vi "Performance Test.vi"() -> ()   [LabVIEW 2021]
uses:
  <vilib>/Platform/TimedLoop/XDataNode/timing_clust.ctl
  <vilib>/Platform/TimedLoop/XDataNode/nitl_modes.ctl
  <vilib>/Platform/TimedLoop/XDataNode/wakeup.ctl
  1483eb5a-b5ac-4c0e-b74c-86c7137b2fd6.vi
  12cff863-7c17-483c-86ff-8b13899d7475.vi
  e1d05524-1b70-4109-b7da-ed5891de264b.vi
  929446f6-8a14-498e-9777-57eb22ff0df0.vi
  225441bf-869c-4d3f-a299-9c2de2de7507.vi
  b5d6512a-7382-4e79-b500-a81ead5716f2.vi
  eb2f4adc-c9c5-4356-9fb7-2e53ab499b8d.vi
  07197f74-83c7-460d-bb9d-2f7d38ffd2b9.vi
  21ba3f00-3ca1-4894-b9dd-4e112eabbaa9.vi
  def0a351-4179-4148-9177-b840eaa38f15.vi
  628c775d-4bce-4786-9b92-72b6beaba665.vi
  f43c1be1-ffa2-434e-887c-5abbb6a0f76a.vi
  b8af7206-5871-4d3b-9378-5cfe84a082f3.vi
  c2d7da70-2e27-4f49-958b-30f48dc9c665.vi
  ac27c80e-df74-46b0-978f-8f0f89081651.vi
  1483eb5a-b5ac-4c0e-b74c-86c7137b2fd6.vi/bd07d5d9-1209-45ad-b636-9e9ab86132fb.vi
  SubVIs/Check Error.vi
  SubVIs/Get dll Path.vi
  SubVIs/Get Element Write Position.vi
  SubVIs/Notify Of New Write.vi
  SubVIs/Wait For N Elements Available.vi
  SubVIs/Get Element Read Position.vi
  SubVIs/Set Element Read Position.vi
  225441bf-869c-4d3f-a299-9c2de2de7507.vi/49b3dd2d-4579-4089-b72e-3f0875c862f2.vi
  21ba3f00-3ca1-4894-b9dd-4e112eabbaa9.vi/49b3dd2d-4579-4089-b72e-3f0875c862f2.vi
  f43c1be1-ffa2-434e-887c-5abbb6a0f76a.vi/49b3dd2d-4579-4089-b72e-3f0875c862f2.vi
  <vilib>/Utility/error.llb/Trim Whitespace.vi
  <vilib>/string/Create NI GUID.vi
  SubVIs/Get Element Description Variant.vi
  <vilib>/Utility/error.llb/Error Cluster From Error Code.vi
  SubVIs/Get Element Info Variant.vi
  <vilib>/Platform/TimedLoop/XDataNode/XDataNode.xnode
  <vilib>/Platform/TimedLoop/XDataNode/XDNodeRunTimeDep.lvlib
  CIF_NI_CIPC.lvlib
panel:
  out "avg write double":dbl
  out "max write double":dbl
  out "avg read double no writer":dbl
  out "max read double no writer":dbl
  out "avg read double":dbl
  out "max read double":dbl
  in  "stop":bool
  out "avg read large array":dbl
  out "max read large array":dbl
  out "pass":bool
  out "error out":errorcluster
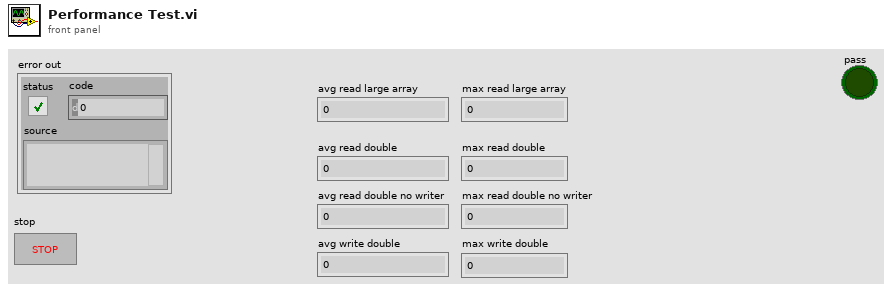
[diagram p1: front panel]
types:
  T1 = typedef "XDNodeRunTimeDep.lvlib/timing_clust.ctl" = cluster{"Expected End [f-1]":u64, "Actual End [f-1]":u64, "Finished Late? [f-1]":bool, "Expected End [i-1]":u64, "Actual End [i-1]":u64, "Finished Late? [i-1]":bool, "Expected Start [i]":u64, "Actual Start [i]":u64, "Expected Start [f]":u64, "Actual Start [f]":u64, "Source Name":string, "Structure Name":string, "Period":i64, "Deadline":i64, "Offset":i64, "Start":i64, "Priority":i32, "Timeout":i32, "Mode":T2, "Wakeup Reason":T3, "Error":errorcluster, "Source Type":string, "Secondary Source Type":string, "Global End Time":u64, "Global Start Time":u64, "Frame Duration":u64, "Iteration Duration":u64, "Assigned CPU":i32, "I/O Scan Engine Mode":u32}
  T2 = typedef "XDNodeRunTimeDep.lvlib/nitl_modes.ctl" = enum32{"No Change", "Process missed periods, maintain original phase", "Discard missed periods, maintain original phase", "Process missed periods, ignore original phase", "Discard missed periods, ignore original phase"}
  T3 = typedef "XDNodeRunTimeDep.lvlib/wakeup.ctl" = enum32{"Normal", "Aborted", "Asynchronous wakeup", "Timing source error", "Timed loop error", "Timeout"}
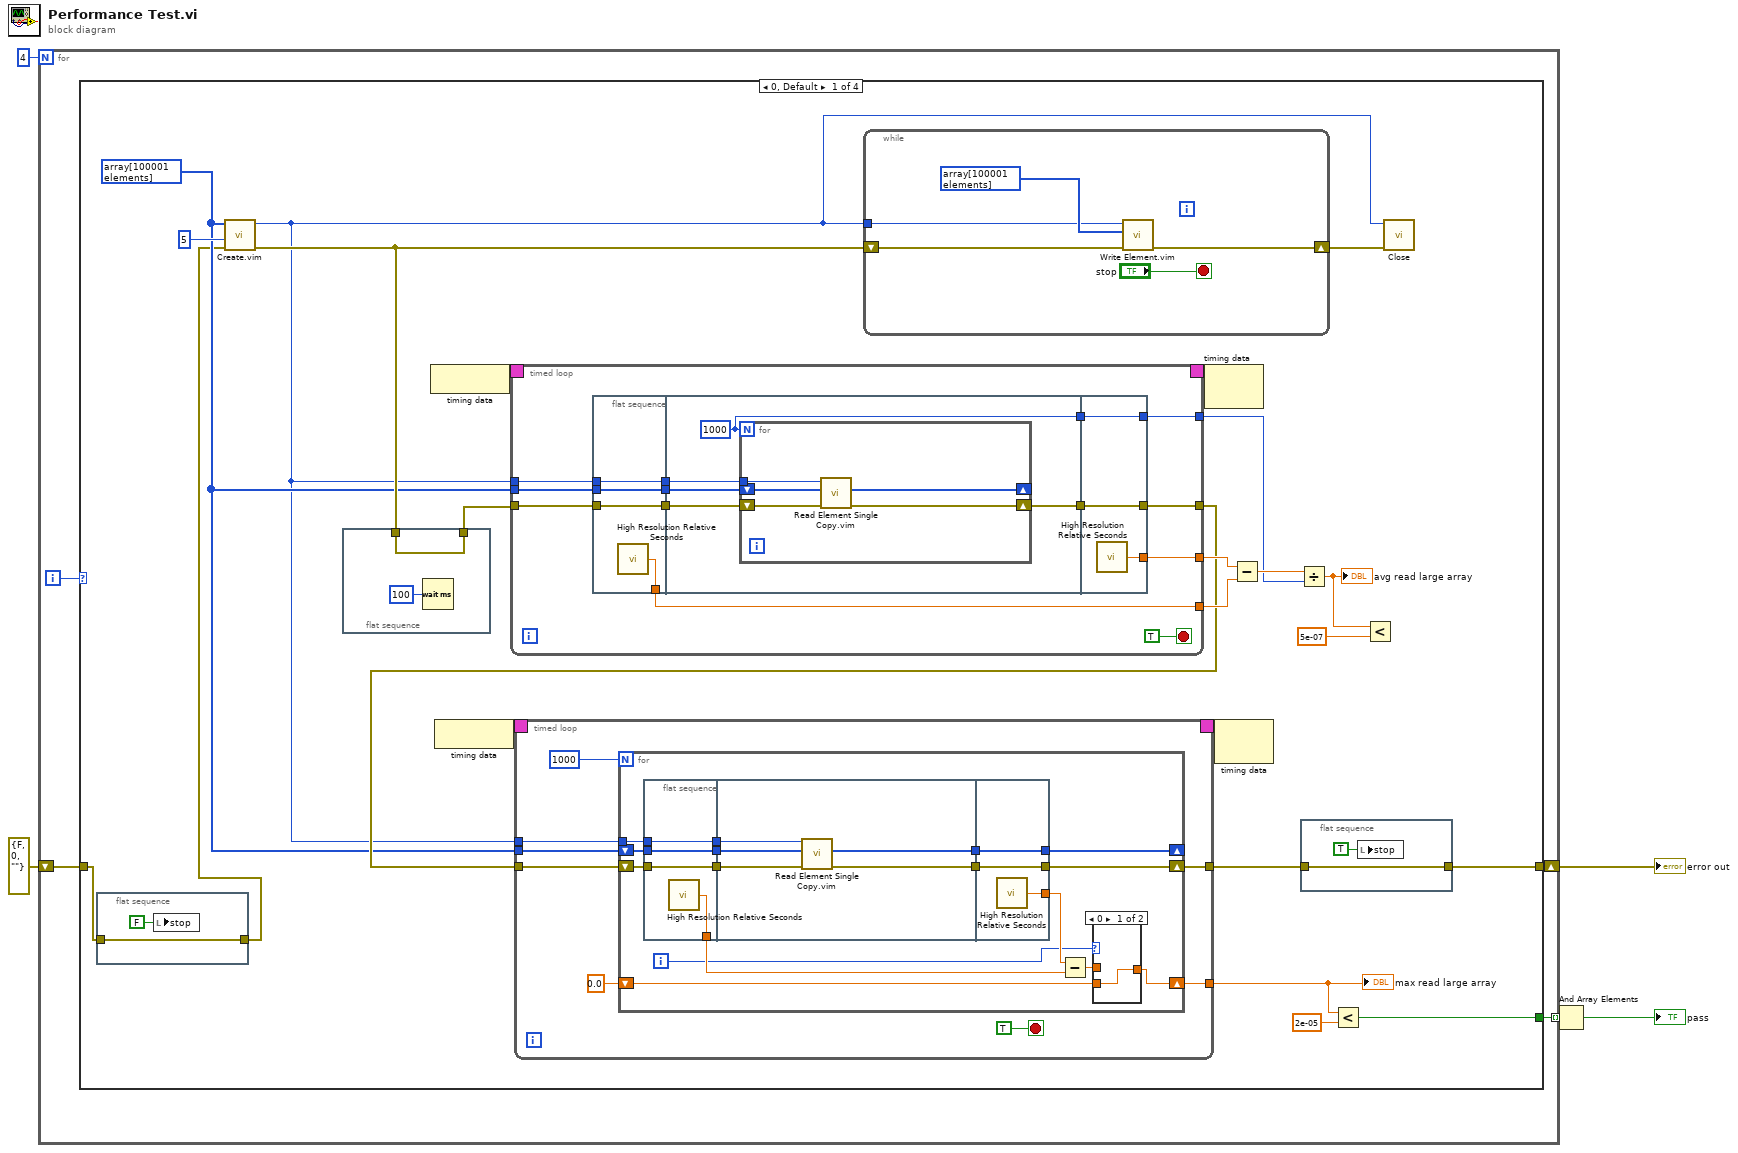
[diagram p0: block diagram]
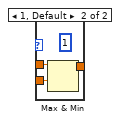
[diagram p2: hidden frame]
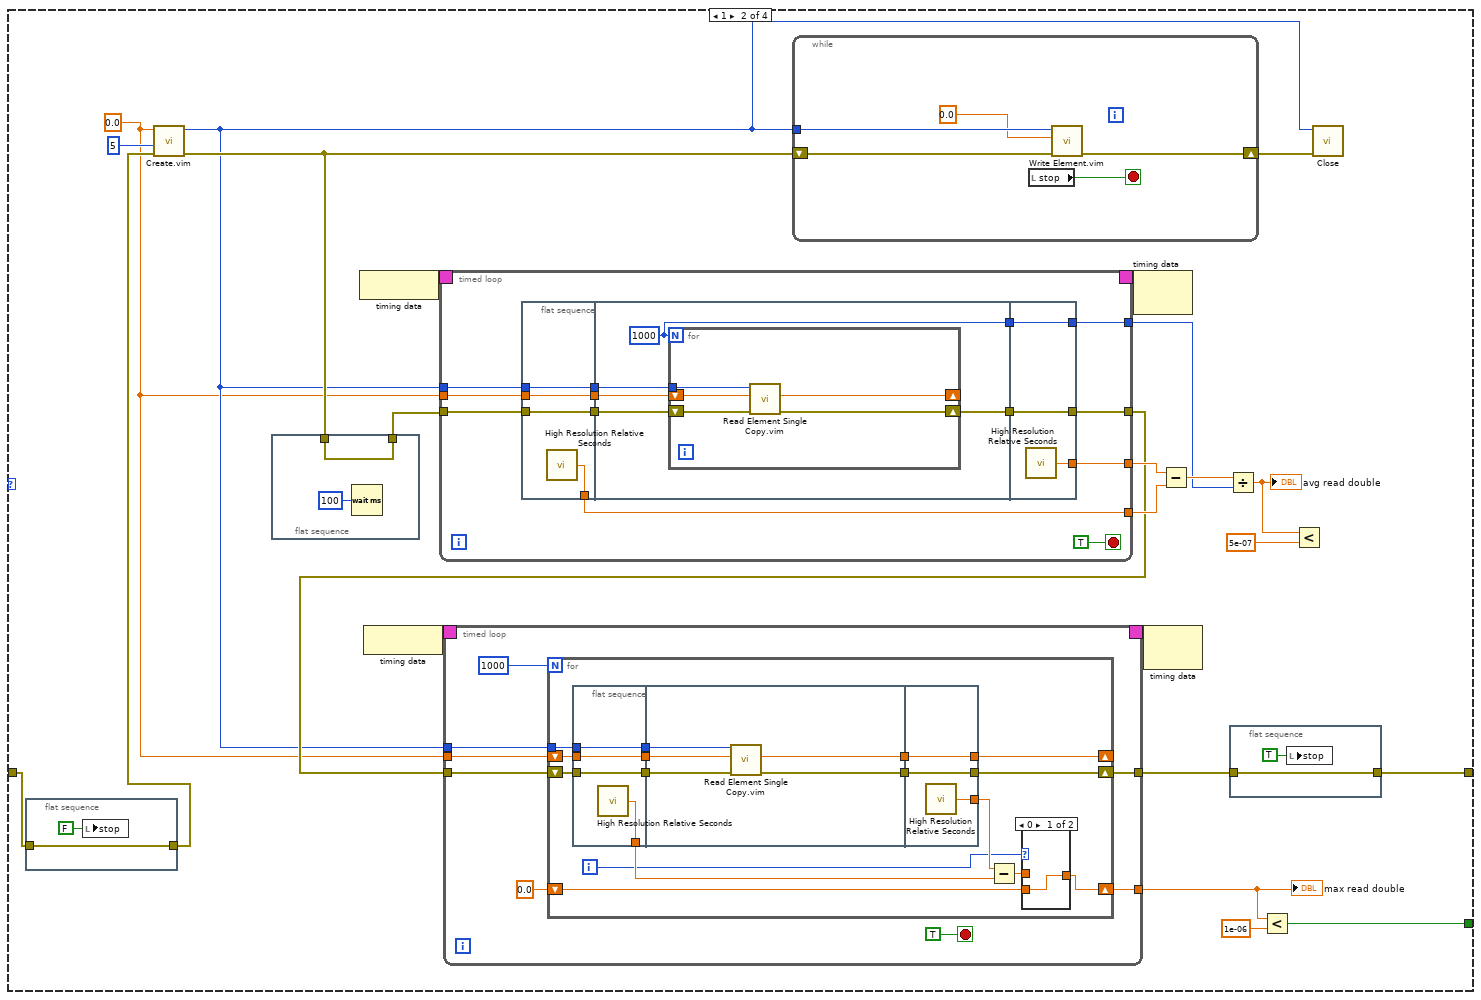
[diagram p3: hidden frame]
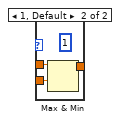
[diagram p4: hidden frame]
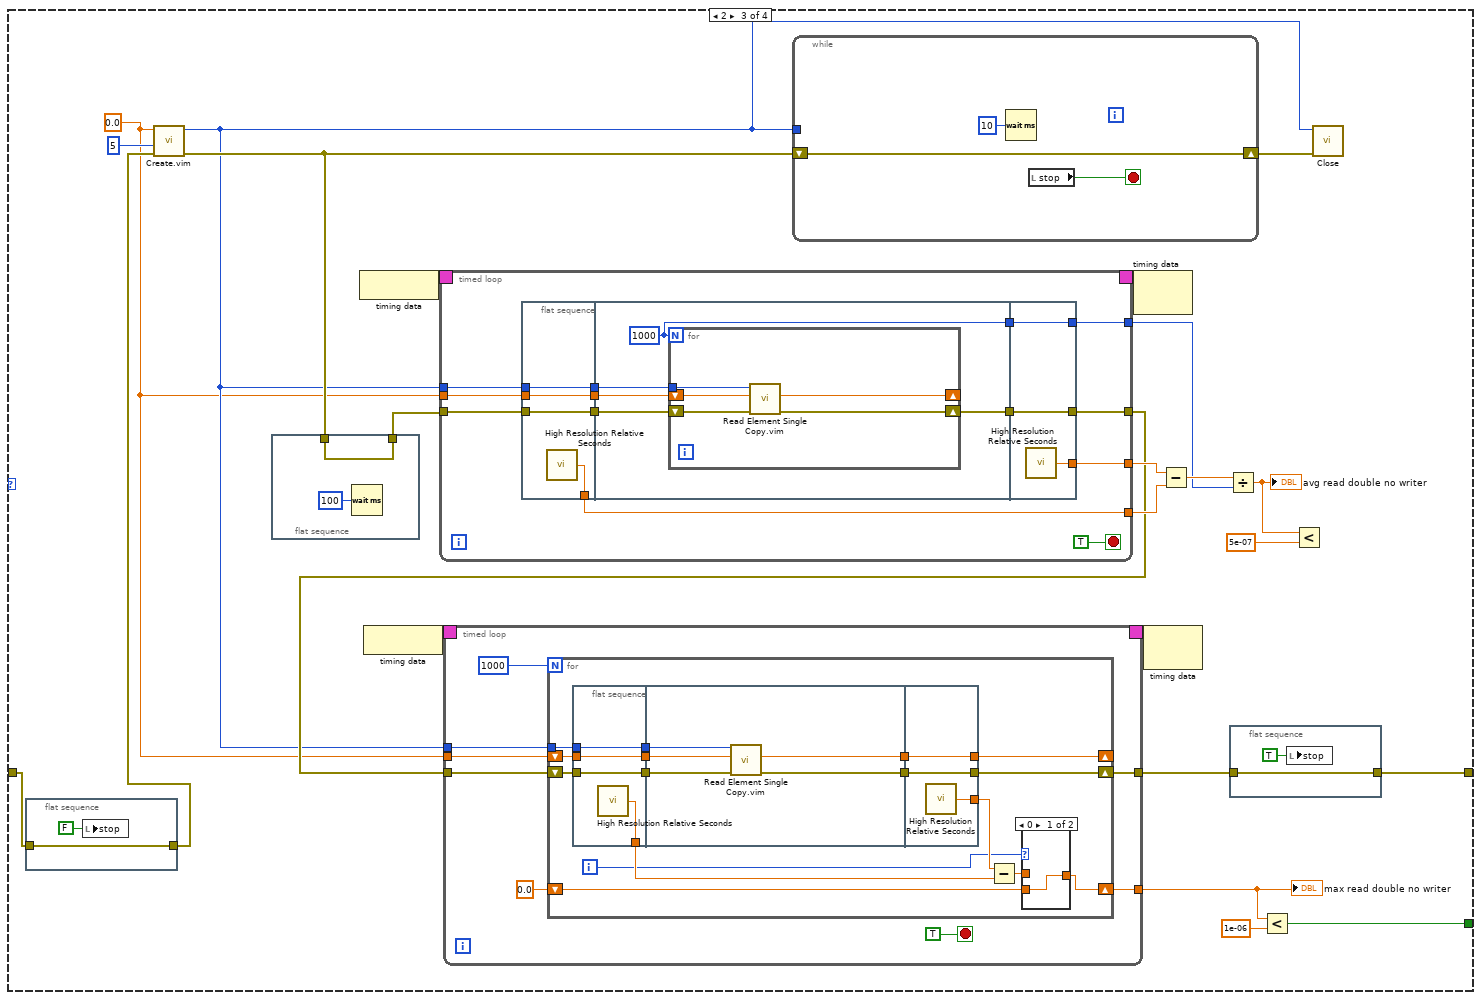
[diagram p5: hidden frame]
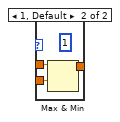
[diagram p6: hidden frame]
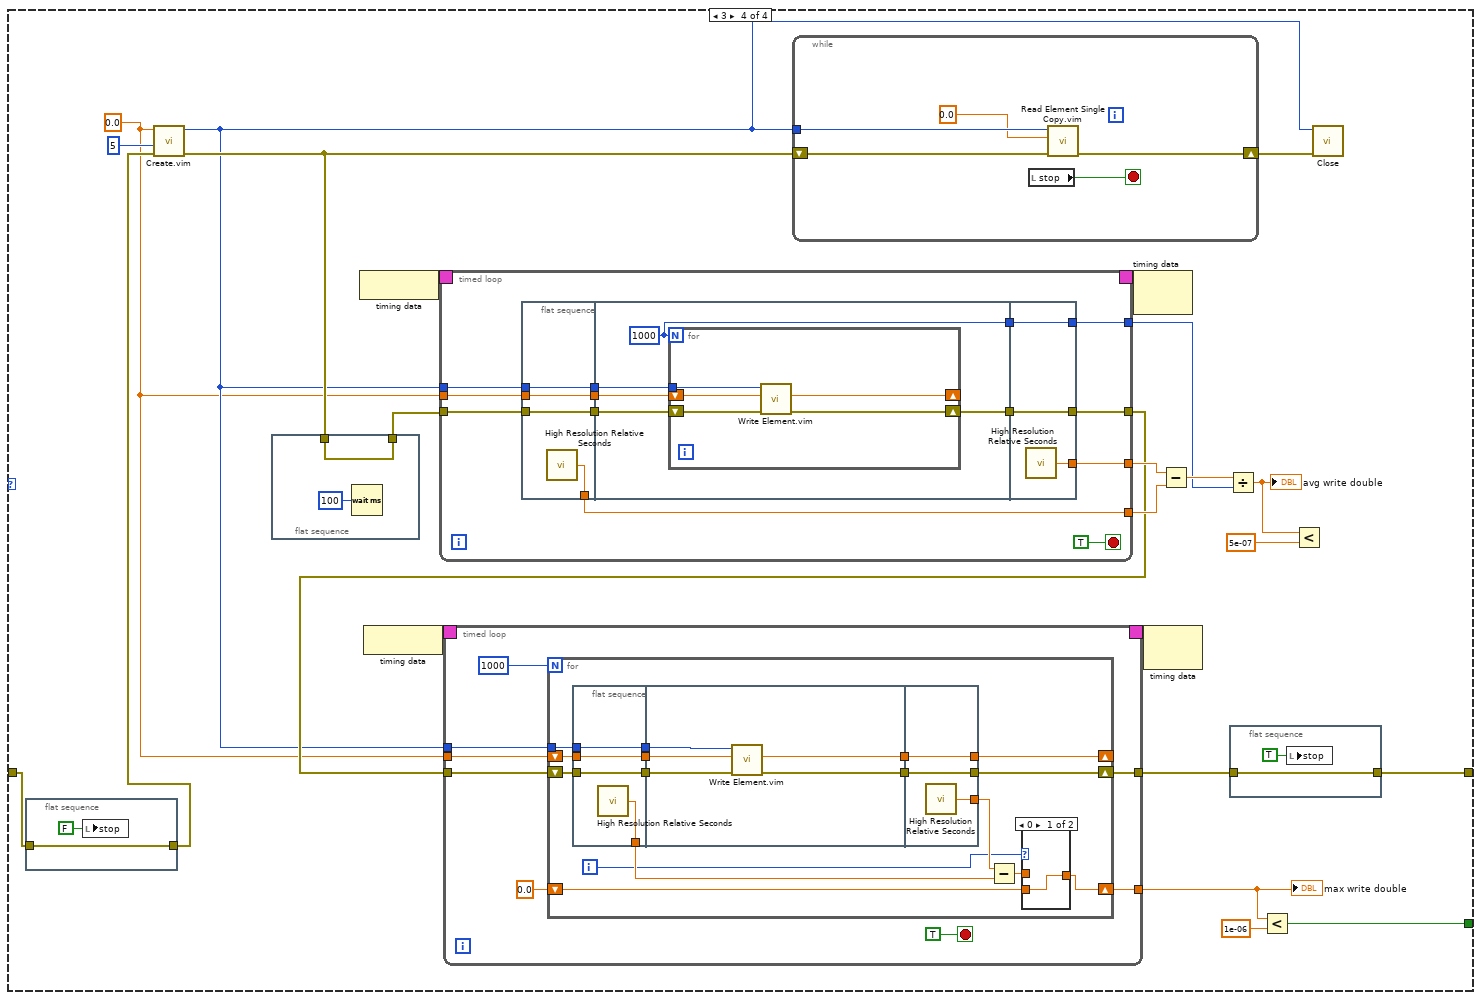
[diagram p7: hidden frame]
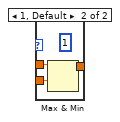
[diagram p8: hidden frame]
diagram:
  n1 = for {
    N: 4 -> [_]
    tunnel: [w9] -> w3 mode=indexing
    shift-right: [w8] -> w5
    shift-left: errorcluster {"status"=FALSE, "code"=0, "source"=""} ("error out") -> [w6]
    i -> [w7]
    n2 = case shown="0, Default" w7 {
      tunnel: [w20 w133 w246 w357] -> w9
      tunnel: [w12 w126 w239 w350] -> w8
      tunnel: w6 -> [w11 w125 w238 w349]
      frame 0, Default {
        w16 = u8[] array[100001 elements] ("U8 Data")
        n3 = flat-sequence {
          tunnel: w11 -> [w35]
          tunnel: [w35] -> w10
          frame #0 {
            n4 = local write "stop"(FALSE ("stop")) -> ()
          }
        }
        n5 = call "Create.vim"("error in (no error)"=w10, "Buffer Size N (2^N)"=u32 5, "Data Type"=w16) -> ("error out"=w17:errorcluster, "CIPC Reference"=w14:u64)  [unwired: 5 in, 2 out]
        n6 = flat-sequence {
          tunnel: w17 -> [w39]
          tunnel: [w39] -> w19
          frame #0 {
            n7 = Wait (ms)(milliseconds to wait=u32 100) -> ()  [unwired: 1 out]
          }
        }
        n8 = node-c288() -> (w33:T1)
        n9 = node-c288() -> (w31:T1)
        n10 = timed-loop {
          timing: w33 -> [_]
          timing-out: [_] -> w32
          tunnel: w14 -> [w91]
          tunnel: w19 -> [w101]
          tunnel: [w98] -> w25
          tunnel: [w96] -> w29
          tunnel: [w95] -> w28
          tunnel: [w94] -> w26
          tunnel: w16 -> [w89]
          stop <- TRUE stop-if-true
          n11 = flat-sequence {
            tunnel: w101 -> [w105]
            tunnel: [w105] -> w99
            tunnel: [w104] -> w95
            tunnel: [w103] -> w92
            tunnel: w91 -> [w103]
            tunnel: [w102] -> w90
            tunnel: w89 -> [w102]
            tunnel: w99 -> [w110]
            tunnel: [w109] -> w97
            tunnel: [w108] -> w93
            tunnel: w92 -> [w107]
            tunnel: w90 -> [w106]
            tunnel: [w118] -> w98
            tunnel: w97 -> [w118]
            tunnel: [w117] -> w96
            tunnel: [w116] -> w94
            tunnel: w93 -> [w116]
            frame #0 {
              n12 = call <vilib>:"High Resolution Relative Seconds.vi"() -> ("relative seconds"=w104:dbl)
            }
            frame #1 {
              w108 = 1000
              n13 = for {
                N: w108 -> [_]
                shift-right: [w113] -> _
                shift-left: w106 -> [w111]
                shift-right: [w114] -> w109
                shift-left: w110 -> [w115]
                tunnel: w107 -> [w112]
                n14 = call "Read Element Single Copy.vim"("error in (no error)"=w115, "Data in"=w111, "CIPC Reference"=w112) -> ("error out"=w114:errorcluster, "Data out"=w113:u8[])  [unwired: 5 in, 2 out]
              }
            }
            frame #2 {
              n15 = call <vilib>:"High Resolution Relative Seconds.vi"() -> ("relative seconds"=w117:dbl)
            }
          }
        }
        n16 = timed-loop {
          timing: w31 -> [_]
          timing-out: [_] -> w30
          tunnel: w25 -> [w52]
          tunnel: [w50] -> w13
          tunnel: [w47] -> w22
          tunnel: w16 -> [w46]
          tunnel: w14 -> [w45]
          stop <- TRUE stop-if-true
          n17 = for {
            N: 1000 -> [_]
            shift-right: [w63] -> _
            shift-left: w46 -> [w65]
            shift-right: [w62] -> w50
            shift-left: w52 -> [w64]
            shift-right: [w57] -> w47
            shift-left: 0.0 -> [w58]
            tunnel: w45 -> [w53]
            i -> [w56]
            n18 = flat-sequence {
              tunnel: w64 -> [w75]
              tunnel: w65 -> [w76]
              tunnel: [w76] -> w68
              tunnel: [w75] -> w67
              tunnel: [w74] -> w60
              tunnel: [w73] -> w54
              tunnel: w53 -> [w73]
              tunnel: w68 -> [w81]
              tunnel: w67 -> [w80]
              tunnel: [w79] -> w66
              tunnel: [w77] -> w55
              tunnel: w54 -> [w78]
              tunnel: [w84] -> w63
              tunnel: w66 -> [w84]
              tunnel: [w83] -> w62
              tunnel: [w82] -> w61
              tunnel: w55 -> [w83]
              frame #0 {
                n19 = call <vilib>:"High Resolution Relative Seconds.vi"() -> ("relative seconds"=w74:dbl)
              }
              frame #1 {
                n20 = call "Read Element Single Copy.vim"("error in (no error)"=w80, "Data in"=w81, "CIPC Reference"=w78) -> ("error out"=w77:errorcluster, "Data out"=w79:u8[])  [unwired: 5 in, 2 out]
              }
              frame #2 {
                n21 = call <vilib>:"High Resolution Relative Seconds.vi"() -> ("relative seconds"=w82:dbl)
              }
            }
            n22 = Subtract(x=w61, y=w60) -> (x-y=w59:dbl)
            n23 = case shown="0" w56 {
              tunnel: w59 -> [_ w72]
              tunnel: w58 -> [w69 w71]
              tunnel: [w69 w70] -> w57
              frame 0 {
              }
              frame 1, Default {
                (unwired) u32 1 ("milliseconds to wait")
                n24 = Max & Min(x=w72, y=w71) -> (max(x,y)=w70:dbl)  [unwired: 1 out]
              }
            }
          }
        }
        "max read large array" <- w22
        n25 = while {
          shift-right: [w43] -> w15
          shift-left: w17 -> [w44]
          tunnel: w14 -> [w41]
          stop <- "stop" stop-if-true
          n26 = call "Write Element.vim"("error in (no error)"=w44, "element"=u8[] array[100001 elements] ("U8 Data"), "CIPC Reference"=w41) -> ("error out"=w43:errorcluster)  [unwired: 6 in, 2 out]
        }
        n27 = node-c288(w32) -> ()  [unwired: 1 out]
        n28 = node-c288(w30) -> ()  [unwired: 1 out]
        n29 = Subtract(x=w29, y=w28) -> (x-y=w27:dbl)
        n30 = Divide(x=w27, y=w26) -> (x/y=w24:dbl)
        "avg read large array" <- w24
        n31 = flat-sequence {
          tunnel: w13 -> [w37]
          tunnel: [w37] -> w12
          frame #0 {
            n32 = local write "stop"(TRUE ("stop")) -> ()
          }
        }
        n33 = Less?(x=w22, y=2e-05) -> (x < y?=w20:bool)
        n34 = Less?(x=w24, y=5e-07) -> ()  [unwired: 1 out]
        n35 = call "Close.vi"("error in (no error)"=w15, "CIPC Reference"=w14) -> ()  [unwired: 9 in, 1 out]
      }
      frame 1 {
        w123 = 0.0
        n36 = flat-sequence {
          tunnel: w125 -> [w148]
          tunnel: [w148] -> w124
          frame #0 {
            n37 = local write "stop"(FALSE ("stop")) -> ()
          }
        }
        n38 = call "Create.vim"("error in (no error)"=w124, "Buffer Size N (2^N)"=u32 5, "Data Type"=w123) -> ("error out"=w130:errorcluster, "CIPC Reference"=w128:u64)  [unwired: 5 in, 2 out]
        n39 = flat-sequence {
          tunnel: w130 -> [w152]
          tunnel: [w152] -> w132
          frame #0 {
            n40 = Wait (ms)(milliseconds to wait=u32 100) -> ()  [unwired: 1 out]
          }
        }
        n41 = node-c288() -> (w146:T1)
        n42 = node-c288() -> (w144:T1)
        n43 = timed-loop {
          timing: w146 -> [_]
          timing-out: [_] -> w145
          tunnel: w128 -> [w204]
          tunnel: w132 -> [w214]
          tunnel: [w211] -> w138
          tunnel: [w209] -> w142
          tunnel: [w208] -> w141
          tunnel: [w207] -> w139
          tunnel: w123 -> [w202]
          stop <- TRUE stop-if-true
          n44 = flat-sequence {
            tunnel: w214 -> [w218]
            tunnel: [w218] -> w212
            tunnel: [w217] -> w208
            tunnel: [w216] -> w205
            tunnel: w204 -> [w216]
            tunnel: [w215] -> w203
            tunnel: w202 -> [w215]
            tunnel: w212 -> [w223]
            tunnel: [w222] -> w210
            tunnel: [w221] -> w206
            tunnel: w205 -> [w220]
            tunnel: w203 -> [w219]
            tunnel: [w231] -> w211
            tunnel: w210 -> [w231]
            tunnel: [w230] -> w209
            tunnel: [w229] -> w207
            tunnel: w206 -> [w229]
            frame #0 {
              n45 = call <vilib>:"High Resolution Relative Seconds.vi"() -> ("relative seconds"=w217:dbl)
            }
            frame #1 {
              w221 = 1000
              n46 = for {
                N: w221 -> [_]
                shift-right: [w226] -> _
                shift-left: w219 -> [w224]
                shift-right: [w227] -> w222
                shift-left: w223 -> [w228]
                tunnel: w220 -> [w225]
                n47 = call "Read Element Single Copy.vim"("error in (no error)"=w228, "Data in"=w224, "CIPC Reference"=w225) -> ("error out"=w227:errorcluster, "Data out"=w226:dbl)  [unwired: 5 in, 2 out]
              }
            }
            frame #2 {
              n48 = call <vilib>:"High Resolution Relative Seconds.vi"() -> ("relative seconds"=w230:dbl)
            }
          }
        }
        n49 = timed-loop {
          timing: w144 -> [_]
          timing-out: [_] -> w143
          tunnel: w138 -> [w165]
          tunnel: [w163] -> w127
          tunnel: [w160] -> w135
          tunnel: w123 -> [w159]
          tunnel: w128 -> [w158]
          stop <- TRUE stop-if-true
          n50 = for {
            N: 1000 -> [_]
            shift-right: [w176] -> _
            shift-left: w159 -> [w178]
            shift-right: [w175] -> w163
            shift-left: w165 -> [w177]
            shift-right: [w170] -> w160
            shift-left: 0.0 -> [w171]
            tunnel: w158 -> [w166]
            i -> [w169]
            n51 = flat-sequence {
              tunnel: w177 -> [w188]
              tunnel: w178 -> [w189]
              tunnel: [w189] -> w181
              tunnel: [w188] -> w180
              tunnel: [w187] -> w173
              tunnel: [w186] -> w167
              tunnel: w166 -> [w186]
              tunnel: w181 -> [w194]
              tunnel: w180 -> [w193]
              tunnel: [w192] -> w179
              tunnel: [w190] -> w168
              tunnel: w167 -> [w191]
              tunnel: [w197] -> w176
              tunnel: w179 -> [w197]
              tunnel: [w196] -> w175
              tunnel: [w195] -> w174
              tunnel: w168 -> [w196]
              frame #0 {
                n52 = call <vilib>:"High Resolution Relative Seconds.vi"() -> ("relative seconds"=w187:dbl)
              }
              frame #1 {
                n53 = call "Read Element Single Copy.vim"("error in (no error)"=w193, "Data in"=w194, "CIPC Reference"=w191) -> ("error out"=w190:errorcluster, "Data out"=w192:dbl)  [unwired: 5 in, 2 out]
              }
              frame #2 {
                n54 = call <vilib>:"High Resolution Relative Seconds.vi"() -> ("relative seconds"=w195:dbl)
              }
            }
            n55 = Subtract(x=w174, y=w173) -> (x-y=w172:dbl)
            n56 = case shown="0" w169 {
              tunnel: w172 -> [_ w185]
              tunnel: w171 -> [w182 w184]
              tunnel: [w182 w183] -> w170
              frame 0 {
              }
              frame 1, Default {
                (unwired) u32 1 ("milliseconds to wait")
                n57 = Max & Min(x=w185, y=w184) -> (max(x,y)=w183:dbl)  [unwired: 1 out]
              }
            }
          }
        }
        "max read double" <- w135
        n58 = while {
          shift-right: [w156] -> w129
          shift-left: w130 -> [w157]
          tunnel: w128 -> [w155]
          stop <- w153 stop-if-true
          n59 = local read "stop"() -> (w153:bool)
          n60 = call "Write Element.vim"("error in (no error)"=w157, "element"=0.0, "CIPC Reference"=w155) -> ("error out"=w156:errorcluster)  [unwired: 6 in, 2 out]
        }
        n61 = node-c288(w145) -> ()  [unwired: 1 out]
        n62 = node-c288(w143) -> ()  [unwired: 1 out]
        n63 = Subtract(x=w142, y=w141) -> (x-y=w140:dbl)
        n64 = Divide(x=w140, y=w139) -> (x/y=w137:dbl)
        "avg read double" <- w137
        n65 = flat-sequence {
          tunnel: w127 -> [w150]
          tunnel: [w150] -> w126
          frame #0 {
            n66 = local write "stop"(TRUE ("stop")) -> ()
          }
        }
        n67 = Less?(x=w135, y=1e-06) -> (x < y?=w133:bool)
        n68 = Less?(x=w137, y=5e-07) -> ()  [unwired: 1 out]
        n69 = call "Close.vi"("error in (no error)"=w129, "CIPC Reference"=w128) -> ()  [unwired: 9 in, 1 out]
      }
      frame 2 {
        w236 = 0.0
        n70 = flat-sequence {
          tunnel: w238 -> [w261]
          tunnel: [w261] -> w237
          frame #0 {
            n71 = local write "stop"(FALSE ("stop")) -> ()
          }
        }
        n72 = call "Create.vim"("error in (no error)"=w237, "Buffer Size N (2^N)"=u32 5, "Data Type"=w236) -> ("error out"=w243:errorcluster, "CIPC Reference"=w241:u64)  [unwired: 5 in, 2 out]
        n73 = flat-sequence {
          tunnel: w243 -> [w265]
          tunnel: [w265] -> w245
          frame #0 {
            n74 = Wait (ms)(milliseconds to wait=u32 100) -> ()  [unwired: 1 out]
          }
        }
        n75 = node-c288() -> (w259:T1)
        n76 = node-c288() -> (w257:T1)
        n77 = timed-loop {
          timing: w259 -> [_]
          timing-out: [_] -> w258
          tunnel: w241 -> [w315]
          tunnel: w245 -> [w325]
          tunnel: [w322] -> w251
          tunnel: [w320] -> w255
          tunnel: [w319] -> w254
          tunnel: [w318] -> w252
          tunnel: w236 -> [w313]
          stop <- TRUE stop-if-true
          n78 = flat-sequence {
            tunnel: w325 -> [w329]
            tunnel: [w329] -> w323
            tunnel: [w328] -> w319
            tunnel: [w327] -> w316
            tunnel: w315 -> [w327]
            tunnel: [w326] -> w314
            tunnel: w313 -> [w326]
            tunnel: w323 -> [w334]
            tunnel: [w333] -> w321
            tunnel: [w332] -> w317
            tunnel: w316 -> [w331]
            tunnel: w314 -> [w330]
            tunnel: [w342] -> w322
            tunnel: w321 -> [w342]
            tunnel: [w341] -> w320
            tunnel: [w340] -> w318
            tunnel: w317 -> [w340]
            frame #0 {
              n79 = call <vilib>:"High Resolution Relative Seconds.vi"() -> ("relative seconds"=w328:dbl)
            }
            frame #1 {
              w332 = 1000
              n80 = for {
                N: w332 -> [_]
                shift-right: [w337] -> _
                shift-left: w330 -> [w335]
                shift-right: [w338] -> w333
                shift-left: w334 -> [w339]
                tunnel: w331 -> [w336]
                n81 = call "Read Element Single Copy.vim"("error in (no error)"=w339, "Data in"=w335, "CIPC Reference"=w336) -> ("error out"=w338:errorcluster, "Data out"=w337:dbl)  [unwired: 5 in, 2 out]
              }
            }
            frame #2 {
              n82 = call <vilib>:"High Resolution Relative Seconds.vi"() -> ("relative seconds"=w341:dbl)
            }
          }
        }
        n83 = timed-loop {
          timing: w257 -> [_]
          timing-out: [_] -> w256
          tunnel: w251 -> [w276]
          tunnel: [w274] -> w240
          tunnel: [w271] -> w248
          tunnel: w236 -> [w270]
          tunnel: w241 -> [w269]
          stop <- TRUE stop-if-true
          n84 = for {
            N: 1000 -> [_]
            shift-right: [w287] -> _
            shift-left: w270 -> [w289]
            shift-right: [w286] -> w274
            shift-left: w276 -> [w288]
            shift-right: [w281] -> w271
            shift-left: 0.0 -> [w282]
            tunnel: w269 -> [w277]
            i -> [w280]
            n85 = flat-sequence {
              tunnel: w288 -> [w299]
              tunnel: w289 -> [w300]
              tunnel: [w300] -> w292
              tunnel: [w299] -> w291
              tunnel: [w298] -> w284
              tunnel: [w297] -> w278
              tunnel: w277 -> [w297]
              tunnel: w292 -> [w305]
              tunnel: w291 -> [w304]
              tunnel: [w303] -> w290
              tunnel: [w301] -> w279
              tunnel: w278 -> [w302]
              tunnel: [w308] -> w287
              tunnel: w290 -> [w308]
              tunnel: [w307] -> w286
              tunnel: [w306] -> w285
              tunnel: w279 -> [w307]
              frame #0 {
                n86 = call <vilib>:"High Resolution Relative Seconds.vi"() -> ("relative seconds"=w298:dbl)
              }
              frame #1 {
                n87 = call "Read Element Single Copy.vim"("error in (no error)"=w304, "Data in"=w305, "CIPC Reference"=w302) -> ("error out"=w301:errorcluster, "Data out"=w303:dbl)  [unwired: 5 in, 2 out]
              }
              frame #2 {
                n88 = call <vilib>:"High Resolution Relative Seconds.vi"() -> ("relative seconds"=w306:dbl)
              }
            }
            n89 = Subtract(x=w285, y=w284) -> (x-y=w283:dbl)
            n90 = case shown="0" w280 {
              tunnel: w283 -> [_ w296]
              tunnel: w282 -> [w293 w295]
              tunnel: [w293 w294] -> w281
              frame 0 {
              }
              frame 1, Default {
                (unwired) u32 1 ("milliseconds to wait")
                n91 = Max & Min(x=w296, y=w295) -> (max(x,y)=w294:dbl)  [unwired: 1 out]
              }
            }
          }
        }
        "max read double no writer" <- w248
        n92 = while {
          shift-right: [w267] -> w242
          shift-left: w243 -> [w267]
          tunnel: w241 -> [_]
          stop <- w268 stop-if-true
          n93 = Wait (ms)(milliseconds to wait=u32 10) -> ()  [unwired: 1 out]
          n94 = local read "stop"() -> (w268:bool)
        }
        n95 = node-c288(w258) -> ()  [unwired: 1 out]
        n96 = node-c288(w256) -> ()  [unwired: 1 out]
        n97 = Subtract(x=w255, y=w254) -> (x-y=w253:dbl)
        n98 = Divide(x=w253, y=w252) -> (x/y=w250:dbl)
        "avg read double no writer" <- w250
        n99 = flat-sequence {
          tunnel: w240 -> [w263]
          tunnel: [w263] -> w239
          frame #0 {
            n100 = local write "stop"(TRUE ("stop")) -> ()
          }
        }
        n101 = Less?(x=w248, y=1e-06) -> (x < y?=w246:bool)
        n102 = Less?(x=w250, y=5e-07) -> ()  [unwired: 1 out]
        n103 = call "Close.vi"("error in (no error)"=w242, "CIPC Reference"=w241) -> ()  [unwired: 9 in, 1 out]
      }
      frame 3 {
        w347 = 0.0
        n104 = flat-sequence {
          tunnel: w349 -> [w372]
          tunnel: [w372] -> w348
          frame #0 {
            n105 = local write "stop"(FALSE ("stop")) -> ()
          }
        }
        n106 = call "Create.vim"("error in (no error)"=w348, "Buffer Size N (2^N)"=u32 5, "Data Type"=w347) -> ("error out"=w354:errorcluster, "CIPC Reference"=w352:u64)  [unwired: 5 in, 2 out]
        n107 = flat-sequence {
          tunnel: w354 -> [w376]
          tunnel: [w376] -> w356
          frame #0 {
            n108 = Wait (ms)(milliseconds to wait=u32 100) -> ()  [unwired: 1 out]
          }
        }
        n109 = node-c288() -> (w370:T1)
        n110 = node-c288() -> (w368:T1)
        n111 = timed-loop {
          timing: w370 -> [_]
          timing-out: [_] -> w369
          tunnel: w352 -> [w428]
          tunnel: w356 -> [w438]
          tunnel: [w435] -> w362
          tunnel: [w433] -> w366
          tunnel: [w432] -> w365
          tunnel: [w431] -> w363
          tunnel: w347 -> [w426]
          stop <- TRUE stop-if-true
          n112 = flat-sequence {
            tunnel: w438 -> [w442]
            tunnel: [w442] -> w436
            tunnel: [w441] -> w432
            tunnel: [w440] -> w429
            tunnel: w428 -> [w440]
            tunnel: [w439] -> w427
            tunnel: w426 -> [w439]
            tunnel: w436 -> [w447]
            tunnel: [w446] -> w434
            tunnel: [w445] -> w430
            tunnel: w429 -> [w444]
            tunnel: w427 -> [w443]
            tunnel: [w455] -> w435
            tunnel: w434 -> [w455]
            tunnel: [w454] -> w433
            tunnel: [w453] -> w431
            tunnel: w430 -> [w453]
            frame #0 {
              n113 = call <vilib>:"High Resolution Relative Seconds.vi"() -> ("relative seconds"=w441:dbl)
            }
            frame #1 {
              w445 = 1000
              n114 = for {
                N: w445 -> [_]
                shift-right: [w449] -> _
                shift-left: w443 -> [w448]
                shift-right: [w450] -> w446
                shift-left: w447 -> [w451]
                tunnel: w444 -> [w452]
                n115 = call "Write Element.vim"("error in (no error)"=w451, "element"=w448, "CIPC Reference"=w452) -> ("error out"=w450:errorcluster, "element_written"=w449:dbl)  [unwired: 6 in, 1 out]
              }
            }
            frame #2 {
              n116 = call <vilib>:"High Resolution Relative Seconds.vi"() -> ("relative seconds"=w454:dbl)
            }
          }
        }
        n117 = timed-loop {
          timing: w368 -> [_]
          timing-out: [_] -> w367
          tunnel: w362 -> [w389]
          tunnel: [w387] -> w351
          tunnel: [w384] -> w359
          tunnel: w347 -> [w383]
          tunnel: w352 -> [w382]
          stop <- TRUE stop-if-true
          n118 = for {
            N: 1000 -> [_]
            shift-right: [w400] -> _
            shift-left: w383 -> [w402]
            shift-right: [w399] -> w387
            shift-left: w389 -> [w401]
            shift-right: [w394] -> w384
            shift-left: 0.0 -> [w395]
            tunnel: w382 -> [w390]
            i -> [w393]
            n119 = flat-sequence {
              tunnel: w401 -> [w412]
              tunnel: w402 -> [w413]
              tunnel: [w413] -> w405
              tunnel: [w412] -> w404
              tunnel: [w411] -> w397
              tunnel: [w410] -> w391
              tunnel: w390 -> [w410]
              tunnel: w405 -> [w415]
              tunnel: w404 -> [w417]
              tunnel: [w414] -> w403
              tunnel: [w416] -> w392
              tunnel: w391 -> [w418]
              tunnel: [w421] -> w400
              tunnel: w403 -> [w421]
              tunnel: [w420] -> w399
              tunnel: [w419] -> w398
              tunnel: w392 -> [w420]
              frame #0 {
                n120 = call <vilib>:"High Resolution Relative Seconds.vi"() -> ("relative seconds"=w411:dbl)
              }
              frame #1 {
                n121 = call "Write Element.vim"("error in (no error)"=w417, "element"=w415, "CIPC Reference"=w418) -> ("error out"=w416:errorcluster, "element_written"=w414:dbl)  [unwired: 6 in, 1 out]
              }
              frame #2 {
                n122 = call <vilib>:"High Resolution Relative Seconds.vi"() -> ("relative seconds"=w419:dbl)
              }
            }
            n123 = Subtract(x=w398, y=w397) -> (x-y=w396:dbl)
            n124 = case shown="0" w393 {
              tunnel: w396 -> [_ w409]
              tunnel: w395 -> [w406 w408]
              tunnel: [w406 w407] -> w394
              frame 0 {
              }
              frame 1, Default {
                (unwired) u32 1 ("milliseconds to wait")
                n125 = Max & Min(x=w409, y=w408) -> (max(x,y)=w407:dbl)  [unwired: 1 out]
              }
            }
          }
        }
        "max write double" <- w359
        n126 = while {
          shift-right: [w379] -> w353
          shift-left: w354 -> [w380]
          tunnel: w352 -> [w378]
          stop <- w381 stop-if-true
          n127 = local read "stop"() -> (w381:bool)
          n128 = call "Read Element Single Copy.vim"("error in (no error)"=w380, "Data in"=0.0, "CIPC Reference"=w378) -> ("error out"=w379:errorcluster)  [unwired: 5 in, 3 out]
        }
        n129 = node-c288(w369) -> ()  [unwired: 1 out]
        n130 = node-c288(w367) -> ()  [unwired: 1 out]
        n131 = Subtract(x=w366, y=w365) -> (x-y=w364:dbl)
        n132 = Divide(x=w364, y=w363) -> (x/y=w361:dbl)
        "avg write double" <- w361
        n133 = flat-sequence {
          tunnel: w351 -> [w374]
          tunnel: [w374] -> w350
          frame #0 {
            n134 = local write "stop"(TRUE ("stop")) -> ()
          }
        }
        n135 = Less?(x=w359, y=1e-06) -> (x < y?=w357:bool)
        n136 = Less?(x=w361, y=5e-07) -> ()  [unwired: 1 out]
        n137 = call "Close.vi"("error in (no error)"=w353, "CIPC Reference"=w352) -> ()  [unwired: 9 in, 1 out]
      }
    }
  }
  "error out" <- w5
  n138 = And Array Elements(Boolean array=w3) -> (logical AND=→"pass":bool)
